vi "Contour Line_Find Candidate Edges (row).vi"(11 "edge":T2) -> (3 "Candidate Edges":T1(array[cluster]))   [LabVIEW 2020, in "NI_AAL_Geometry.lvlib"]
uses:
  <vilib>/Analysis/NI_AAL_Geometry.lvlib
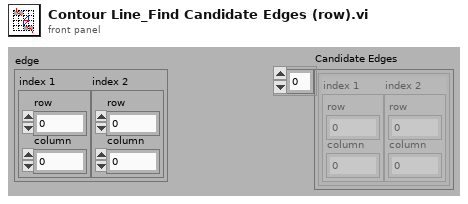
[diagram p1: front panel]
types:
  T1 = cluster{"index 1":cluster{"row":i32, "column":i32}, "index 2":cluster{"row":i32, "column":i32}}[]
  T2 = cluster{"index 1":cluster{"row":i32, "column":i32}, "index 2":cluster{"row":i32, "column":i32}}
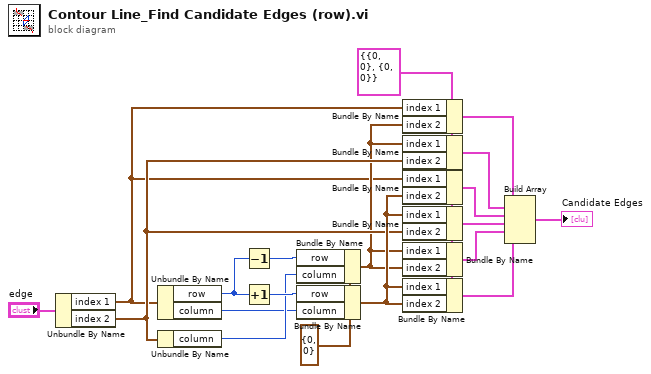
[diagram p0: block diagram]
diagram:
  w14 = cluster{"row":i32, "column":i32} {"row"=0, "column"=0} ("index 2")
  w12 = T2 {"index 1"={"row"=0, "column"=0}, "index 2"={"row"=0, "column"=0}} ("edge")
  n1 = Unbundle By Name("edge") -> ("index 1"=w1:cluster{"row":i32, "column":i32}, "index 2"=w3:cluster{"row":i32, "column":i32})
  n2 = Unbundle By Name(w1) -> ("row"=w17:i32, "column"=w13:i32)
  n3 = Unbundle By Name(w3) -> ("column"=w15:i32)
  n4 = Decrement(x=w17) -> (x-1=w18:i32)
  n5 = Increment(x=w17) -> (x+1=w16:i32)
  n6 = Bundle By Name(cluster=w14, "row"=w18, "column"=w15) -> (w2:cluster{"row":i32, "column":i32})
  n7 = Bundle By Name(cluster=w14, "row"=w16, "column"=w13) -> (w11:cluster{"row":i32, "column":i32})
  n8 = Bundle By Name(cluster=w12, "index 1"=w1, "index 2"=w2) -> (w10:T2)
  n9 = Bundle By Name(cluster=w12, "index 1"=w2, "index 2"=w3) -> (w9:T2)
  n10 = Bundle By Name(cluster=w12, "index 1"=w1, "index 2"=w11) -> (w8:T2)
  n11 = Bundle By Name(cluster=w12, "index 1"=w11, "index 2"=w3) -> (w7:T2)
  n12 = Bundle By Name(cluster=w12, "index 1"=w2, "index 2"=w2) -> (w6:T2)
  n13 = Bundle By Name(cluster=w12, "index 1"=w11, "index 2"=w11) -> (w5:T2)
  n14 = Build Array(w10, w9, w8, w7, w6, w5) -> (→"Candidate Edges":T1)
